vi "路径 Json，XML 扁平化.vi"() -> ()   [LabVIEW 2023]
uses:
  batter.ctl
panel:
  out "unFlatten Json":T1
  out "JSON string":string
  in  "Cluster":T2
  out "error out":errorcluster
  in  "输入数据":string
  in  "access (0:read/write)":enum16{"read/write", "read-only", "write-only"}(ring)
  in  "operation (0:open)":T3(ring)
  in  "file path (use dialog)":path
  # "路径 Json，XML 扁平化"
  # "1。 创建文件，并写入JSON  数据"
  # "/Users/yuxintong"
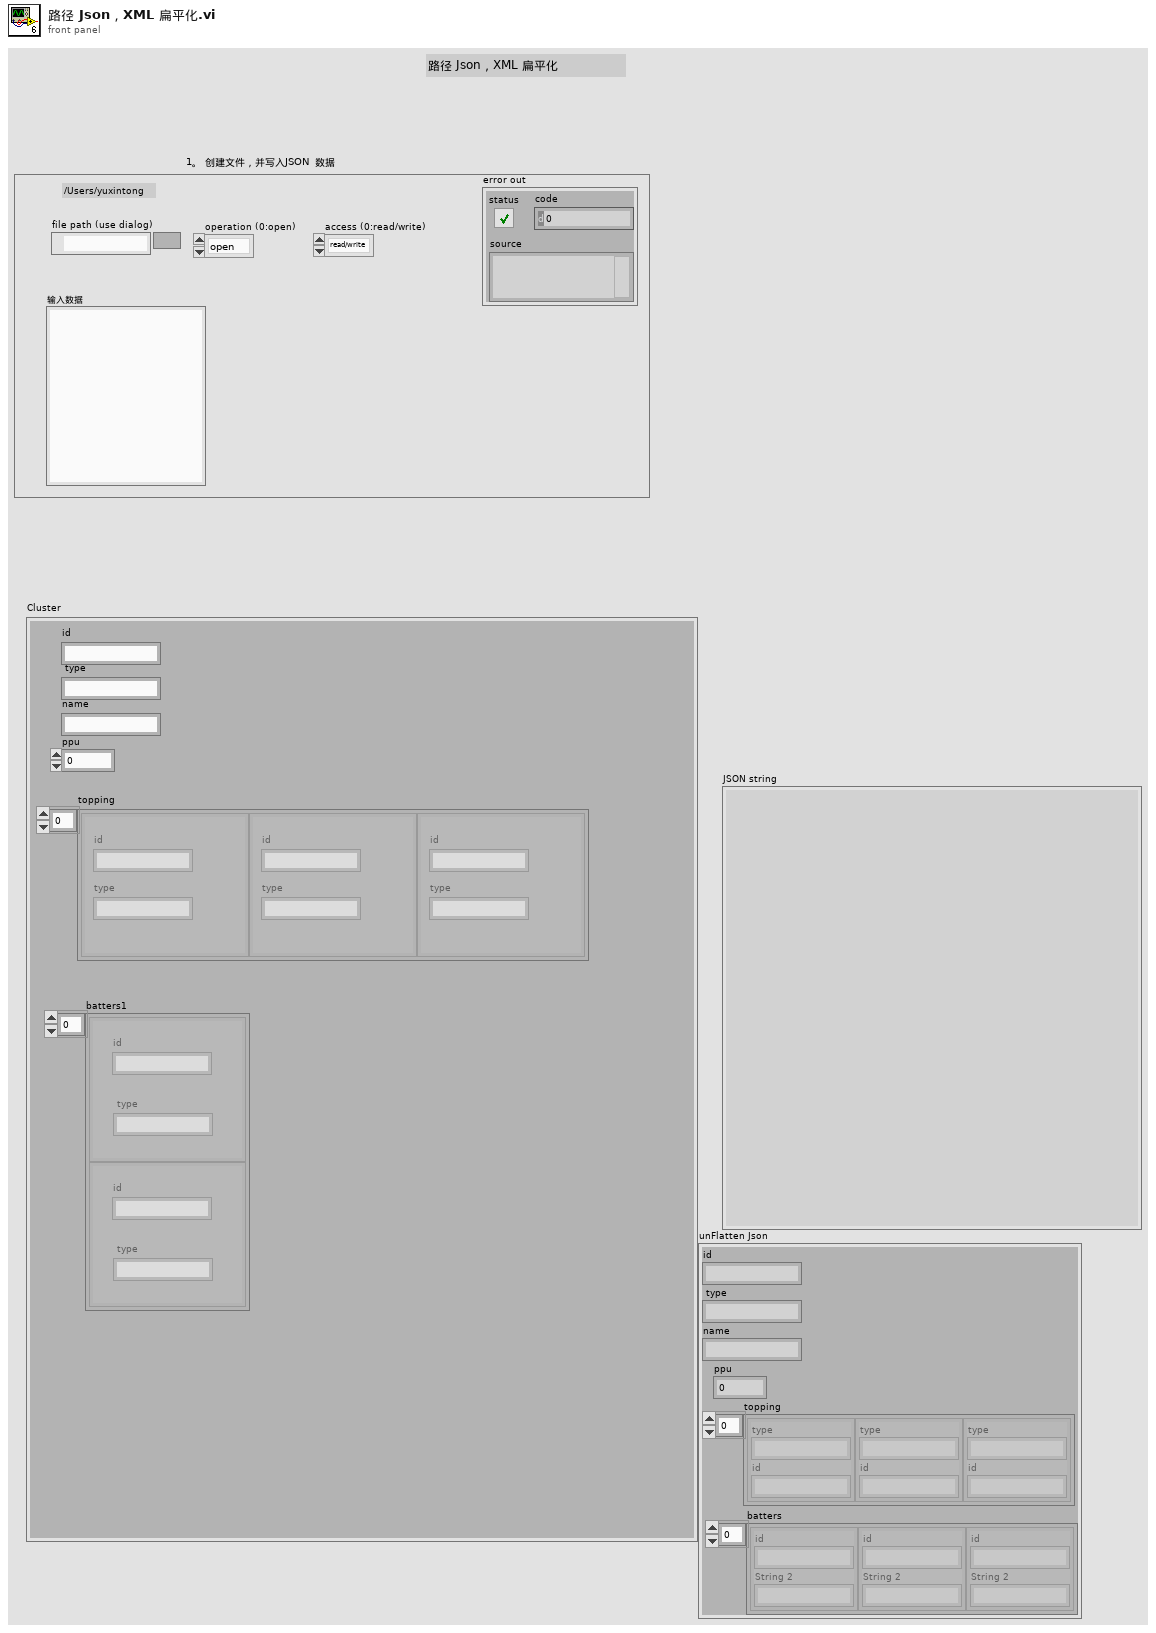
[diagram p1: front panel]
types:
  T1 = cluster{"id":string, " type":string, "name":string, "ppu":dbl, "topping":cluster{"type":string, "id":string}[], "batters":cluster{"id":string, "String 2":string}[]}
  T2 = cluster{"id":string, " type":string, "name":string, "ppu":dbl, "topping":cluster{"type":string, "id":string}[], "batters1":cluster{"id":string, " type":string}[]}
  T3 = enum16{"open", "replace", "create", "open or create", "replace or create", "replace or create with confirmation"}
  T4 = typedef "batter.ctl" = cluster{"id":string, " type":string}[]
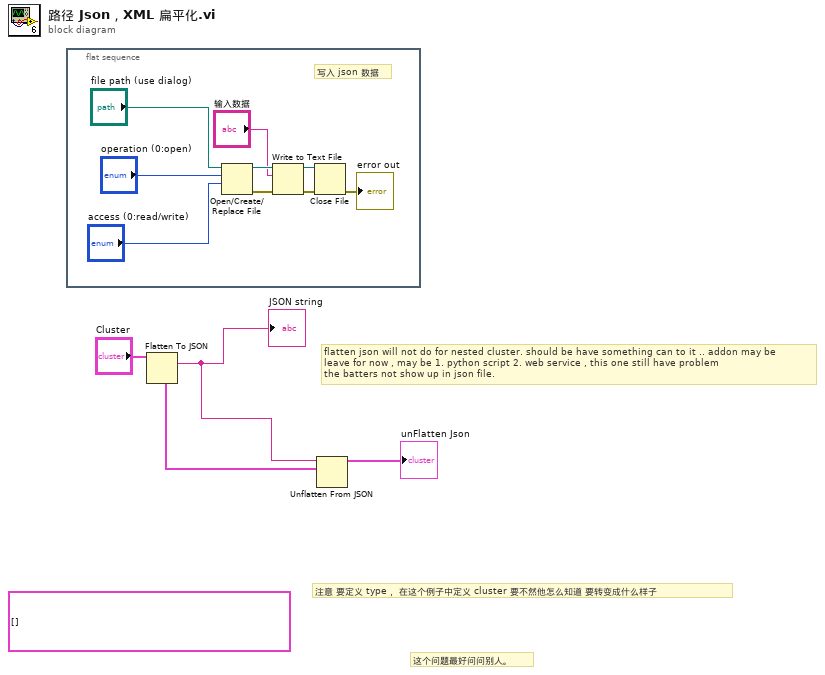
[diagram p0: block diagram]
diagram:
  (unwired) T4 []
  # "这个问题最好问问别人。"
  # "注意 要定义 type， 在这个例子中定义 cluster 要不然他怎么知道 要转变成什么样子"
  # "flatten json will not do for nested cluster. should be have something can to it .. addon may be \nleave for now , may be 1. python script 2. web service , this one still have problem \nthe batters not show up in json file."
  n1 = flat-sequence {
    frame #0 {
      # "写入 json 数据"
      n2 = Open/Create/Replace File(file path (use dialog)="file path (use dialog)", operation (0:open)="operation (0:open)", access (0:read/write)="access (0:read/write)") -> (refnum out=w9:refnum<file>, error out=w8:errorcluster)  [unwired: 3 in, 1 out]
      n3 = Write to Text File(file (use dialog)=w9, text="输入数据", error in=w8) -> (refnum out=w6:refnum<file>, error out=w5:errorcluster)  [unwired: 1 in, 1 out]
      n4 = Close File(refnum=w6, error in=w5) -> (error out=→"error out":errorcluster)  [unwired: 1 out]
    }
  }
  n5 = Flatten To JSON(anything="Cluster") -> (JSON string=w3:string)  [unwired: 2 in, 1 out]
  "JSON string" <- w3
  n6 = Unflatten From JSON(JSON string=w3, type and defaults="Cluster") -> (value=→"unFlatten Json":T2)  [unwired: 5 in, 1 out]
